vi "Read_value_of_earlier_Ch.vi"(3 "Desired Ch to Read":string, 4 "Ch names":string[](array[string]), 5 "Present scan array":dbl[](array[numeric]) format="%.2f") -> (0 "Value":dbl format="%.2f", 1 "Scan comment":string)   [LabVIEW 2010]
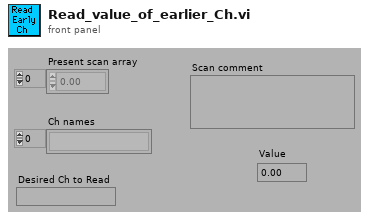
[diagram p1: front panel]
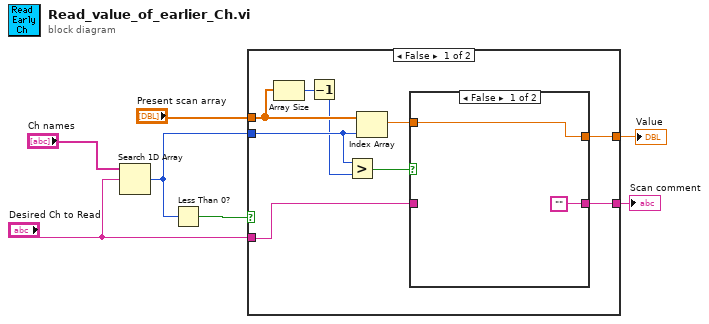
[diagram p0: block diagram]
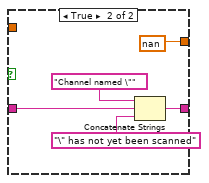
[diagram p2: hidden frame]
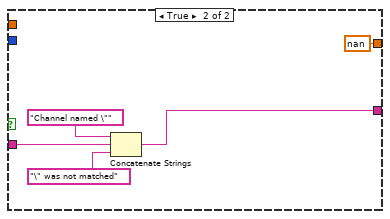
[diagram p3: hidden frame]
diagram:
  n1 = Search 1D Array(1D array="Ch names", element="Desired Ch to Read") -> (index of element=w4:i32)  [unwired: 1 out]
  n2 = Less Than 0?(x=w4) -> (x < 0?=w6:bool)
  n3 = case shown="False" w6 {
    tunnel: "Desired Ch to Read" -> [w11 w26]
    tunnel: "Present scan array" -> [w16 _]
    tunnel: w4 -> [w14 _]
    tunnel: [w10 w25] -> w2
    tunnel: [w9 nan] -> w1
    frame False {
      n4 = Array Size(array=w16) -> (size(s)=w15:i32)
      n5 = Decrement(x=w15) -> (x-1=w13:i32)
      n6 = Greater?(x=w14, y=w13) -> (0:w12:bool)
      n7 = Index Array(array=w16, index=w14) -> (element=w8:dbl)
      n8 = case shown="False" w12 {
        tunnel: w11 -> [_ w21]
        tunnel: ["" w20] -> w10
        tunnel: [w18 nan] -> w9
        tunnel: w8 -> [w18 _]
        frame False {
        }
        frame True {
          n9 = Concatenate Strings("Channel named \"", w21, "\" has not yet been scanned") -> (w20:string)
        }
      }
    }
    frame True {
      n10 = Concatenate Strings("Channel named \"", w26, "\" was not matched") -> (w25:string)
    }
  }
  "Scan comment" <- w2
  "Value" <- w1
